vi "DFT_Compute Average Spectra.vi"(6 "averaging parameters":T2, 8 "error in":errorcluster, 10 "Window":T1 items=["Rectangle"=0, "Hanning"=1, "Hamming"=2, "Blackman-Harris"=3, "Exact Blackman"=4, "Blackman"=5, "Flat Top"=6, "4 Term B-Harris "=7, "7 Term B-Harris"=8, "Low Sidelobe"=9, "Blackman Nuttall"=11, "Triangle"=30, "Bartlett-Hanning"=31, "Bohman"=32, "Parzen"=33, "Welch"=34, "Kaiser"=60, "Dolph-Chebyshev"=61, "Gaussian"=62], 11 "waveforms subset":waveform(dbl)[](array[waveform])) -> (0 "error out":errorcluster, 2 "spectrum info":T3[](array[typedef]) {"x-axis units" items=["Time (s)"=0, "Frequency-CB (Hz)"=1, "Frequency-CPB (Hz)"=1248, "Frequency-Arbitrary (Hz)"=2357, "Quefrency (s)"=2, "Revolutions (rev)"=3, "Order"=4, "Speed (RPM)"=11, "Speed (rad/s)"=21, "Index"=65535]; "weighting filter" items=["Linear", "A-weighting", "B-weighting", "C-weighting", "ITU-R 468-4", "Dolby", "CCITT", "C-message", "Wb", "Wc", "Wd", "We", "Wf", "Wh", "Wj", "Wk", "Wm", "AES17 20 kHz lowpass", "AES17 40 kHz lowpass", "AES17 20 kHz highpass", "AES17 40 kHz highpass"]; "dB reference [EU]" format="%.2f"; "engineering units" items=["custom..."=0, "V"=1, "A"=21, "C"=30, "pC"=31, "s"=32, "-"=29, "Pa"=2, "N"=20, "g"=3, "m/s^2"=4, "m/s"=5, "m"=6, "mm/s"=12, "mm"=13, "micron/s"=14, "micron"=15, "in/s^2"=7, "in/s"=8, "in"=9, "mil/s"=10, "mil"=11, "rad/s^2"=16, "rad/s"=17, "rad"=18, "deg/s^2"=26, "deg/s"=27, "deg"=28, "RPM"=22, "cycle/s^2"=23, "Hz"=24, "cycle"=25, "strain"=19]; "spectral info"."window" items=["None "=0, "Hanning"=1, "Hamming"=2, "Blackman-Harris"=3, "Exact Blackman"=4, "Blackman"=5, "Flat Top"=6, "4 Term B-Harris "=7, "7 Term B-Harris"=8, "Low Sidelobe"=9, "Force - Exponential"=10, "Gaussian"=62]}, 3 "power spectra [dB EU]":cluster{"f0":dbl, "df":dbl, "magnitude":dbl[]}[](array[cluster]), 4 "averages completed":dbl)   [LabVIEW 2024, in "DFT_Spectra.lvlib" / "DFT_Spectra.lvclass"]
uses:
  DFT_Spectra.lvclass
  <vilib>/addons/_NISVFA/_Shared subVIs/Controls/svc_Spectrum Info.ctl
  <vilib>/addons/_NISVFA/_Shared subVIs/Controls/svc_X-Axis Units.ctl
  <vilib>/addons/_NISVFA/_Shared subVIs/Controls/svc_Spectrum Type.ctl
  <vilib>/addons/_NISVFA/_Shared subVIs/Controls/svc_Engineering Units Text Ring.ctl
  <vilib>/addons/_NISVFA/_Shared subVIs/Controls/svc_Weighting Filter Text Ring.ctl
  <vilib>/addons/_NISVFA/_Shared subVIs/Controls/svc_Complimentary Spectrum Units.ctl
  <vilib>/Analysis/4window.llb/windowTd.ctl
  <vilib>/addons/_NISVFA/_Baseband FFT/SVFA Power Spectrum (N Ch).vi
  <vilib>/Analysis/NI_AALPro.lvlib
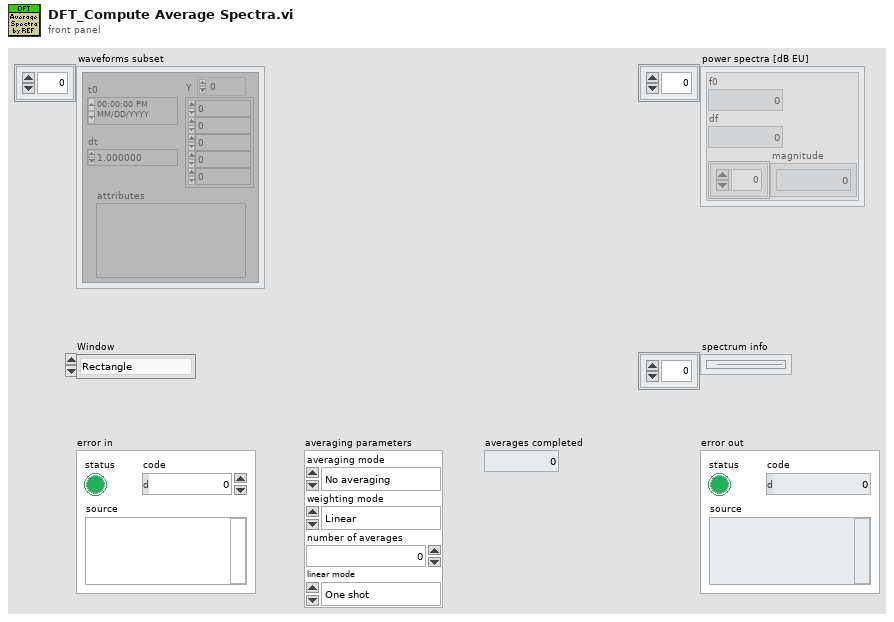
[diagram p1: front panel]
types:
  T1 = typedef "NI_AALPro.lvlib/windowTd.ctl" = u32
  T2 = cluster{"averaging mode":enum16{"No averaging", "Vector averaging", "RMS averaging", "Peak hold"}, "weighting mode":enum16{"Linear", "Exponential"}, "number of averages":u32, "linear mode":enum16{"One shot", "Auto restart"}}
  T3 = typedef "svc_Spectrum Info.ctl" = cluster{"channel name":string, "description":string, "x-axis units":T4, "spectral info":cluster{"spectrum type":T5, "linear/dB":enum16{"linear", "dB"}, "window":u16, "window size":i32, "FFT size":i32}, "engineering units":T6, "custom label":string, "dB reference [EU]":dbl, "peak units":enum16{"rms", "peak", "peak-peak"}, "weighting filter":T7, "spectral density?":bool, "unit label":string, "spectrum skewed?":bool, "complimentary spectrum units":T8}
  T4 = typedef "svc_X-Axis Units.ctl" = u16
  T5 = typedef "svc_Spectrum Type.ctl" = enum16{"FFT Spectrum [complex]", "Amplitude [Magnitude]", "Power [Magnitude^2]", "Cross Spectrum [complex]", "Frequency Response [Complex]"}
  T6 = typedef "svc_Engineering Units Text Ring.ctl" = u16
  T7 = typedef "svc_Weighting Filter Text Ring.ctl" = u16
  T8 = typedef "svc_Complimentary Spectrum Units.ctl" = enum16{"none", "radians", "degrees", "cycles", "imaginary"}
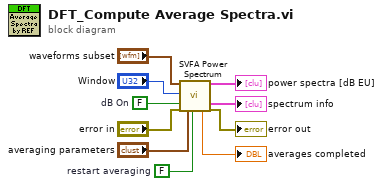
[diagram p0: block diagram]
diagram:
  w1 = FALSE  # restart averaging
  w5 = FALSE  # dB On
  n1 = call-poly <vilib>:"SVFA Power Spectrum.vi"("scaled signals [EU]"="waveforms subset", "window"="Window", "dB On (T)"=w5, "error in (no error)"="error in", "averaging parameters"="averaging parameters", "restart averaging (F)"=w1) -> ("averages completed"=→"averages completed":dbl, "power spectra [dB EU]"=→"power spectra [dB EU]":cluster{"f0":dbl, "df":dbl, "magnitude":dbl[]}[], "spectrum info"=→"spectrum info":T3[], "error out"=→"error out":errorcluster)  [unwired: 8 in, 2 out]
